vi "InitAppearance.vi"(8 "error in (no error)":errorcluster, 9 "Table Ref in":refnum<vi>, 10 "Col #":i32, 11 "Column in":refnum<class "Column.lvclass">) -> (0 "error out":errorcluster, 1 "Table Ref out":refnum<vi>, 3 "Column out":refnum<class "Column.lvclass">)   [LabVIEW 2013, in "Column.lvclass"]
doc: "Set column header, width, background and text color for entire table column."
uses:
  Column.lvclass
  <vilib>/Utility/miscctls.llb/LVRowAndColumnTypeDef.ctl
  Column.lvclass/Column.ctl
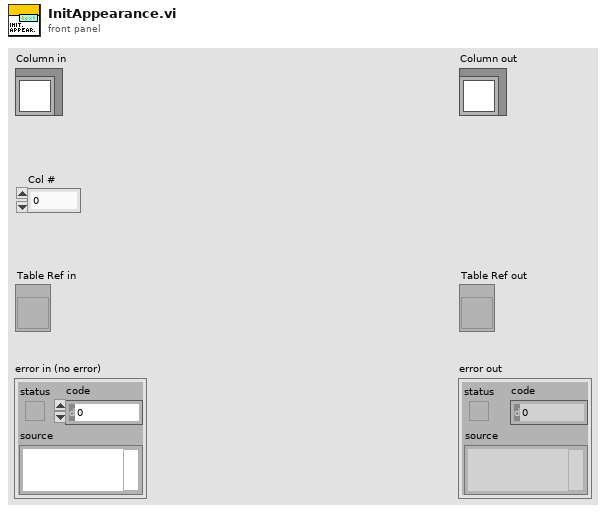
[diagram p1: front panel]
types:
  T1 = typedef "LVRowAndColumnTypeDef.ctl" = cluster{"Row":i32, "Column":i32}
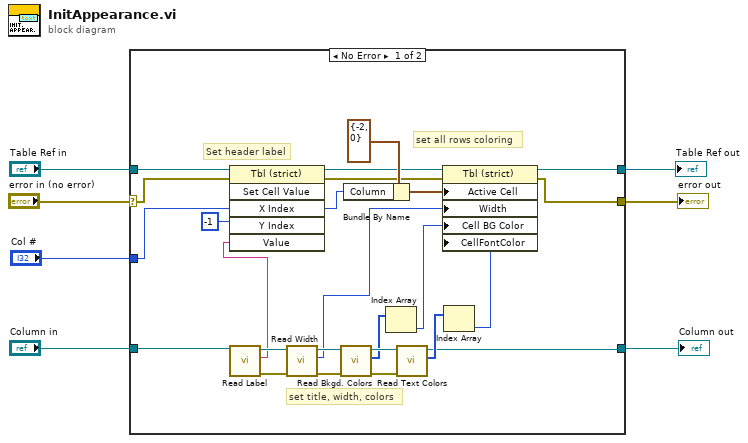
[diagram p0: block diagram]
diagram:
  n1 = case shown="No Error" "error in (no error)" {
    selector: "error in (no error)" -> [w14 w34]
    tunnel: [w15 w34] -> w6
    tunnel: [w11 w33] -> w4
    tunnel: "Column in" -> [w12 w33]
    tunnel: "Table Ref in" -> [w17 w32]
    tunnel: [w16 w32] -> w2
    tunnel: "Col #" -> [w13 _]
    frame No Error {
      # "Set header label"
      # "set title, width, colors"
      # "set all rows coloring"
      n2 = call "Read Label.vi"("Column in"=w12) -> ("error out"=w10:errorcluster, "Label"=w28:string, "Column out"=w31:refnum<class "Column.lvclass">)  [unwired: 8 in]
      n3 = invoke on="Invoke Node" class="Tbl (strict)" method="Set Cell Value"(reference=w17, error in=w14, "X Index"=w13, "Y Index"=-1 ("X Index"), "Value"=w28) -> (reference out=w19:refnum<vi>, error out=w18:errorcluster)  [unwired: 1 in, 4 out]
      n4 = call "Read Width.vi"("error in (no error)"=w10, "Column in"=w31) -> ("error out"=w9:errorcluster, "Width"=w20:u32, "Column out"=w30:refnum<class "Column.lvclass">)  [unwired: 7 in]
      n5 = call "Read Bkgd. Colors.vi"("error in (no error)"=w9, "Column in"=w30) -> ("error out"=w8:errorcluster, "Bkgd. Colors"=w22:u32[], "Column out"=w29:refnum<class "Column.lvclass">)  [unwired: 7 in]
      n6 = Bundle By Name(cluster=T1 {"Row"=-2, "Column"=0} ("RowAndCollumn"), "Column"=w13) -> (w25:T1)
      n7 = Index Array(array=w22) -> (element=w21:u32)  [unwired: 1 in]
      n8 = call "Read Text Colors.vi"("error in (no error)"=w8, "Column in"=w29) -> ("Text Colors"=w24:u32[], "Column out"=w11:refnum<class "Column.lvclass">)  [unwired: 7 in, 1 out]
      n9 = Index Array(array=w24) -> (element=w23:u32)  [unwired: 1 in]
      n10 = property class="Tbl (strict)"(reference=w19, error in=w18, "Active Cell"=w25, "Width"=w20, "Cell BG Color"=w21, "CellFontColor"=w23) -> (reference out=w16:refnum<vi>, error out=w15:errorcluster)
    }
    frame Error {
    }
  }
  "error out" <- w6
  "Column out" <- w4
  "Table Ref out" <- w2
